vi "_CmdExe._Test run VI with abort and timeout.vi"() -> ()   [LabVIEW 2018]
panel:
  out "Timed Out":bool
  out "Aborted":bool
  out "error out":errorcluster
  in  "Timeout ms":i32=2000
  in  "Test Start":bool
  in  "stop":bool
  out "Running":bool
  in  "Abort":bool
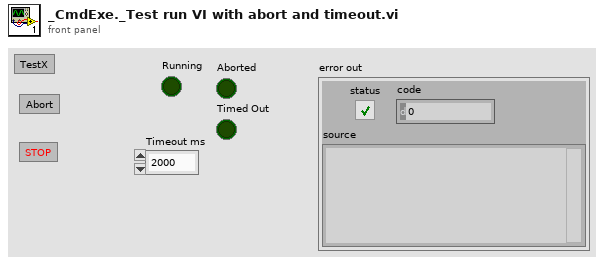
[diagram p1: front panel]
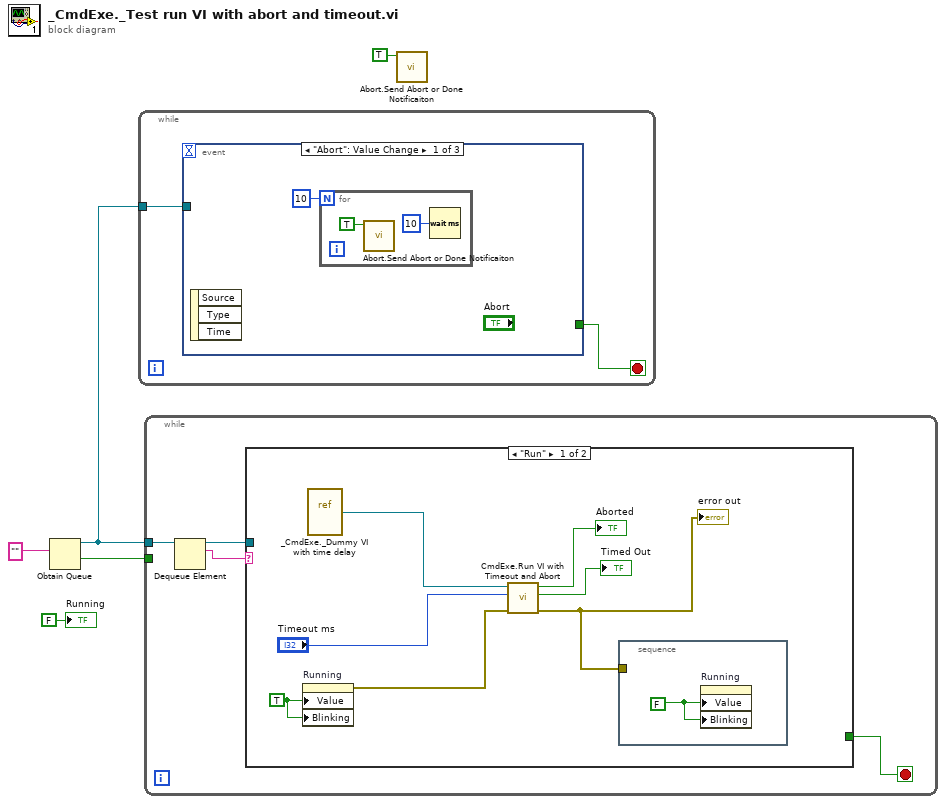
[diagram p0: block diagram]
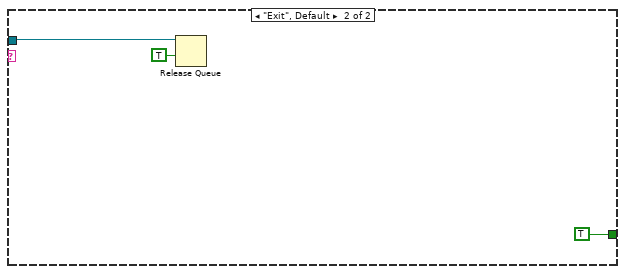
[diagram p2: hidden frame]
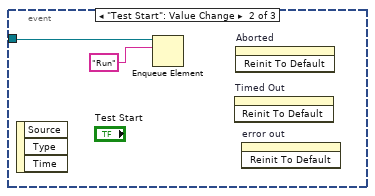
[diagram p3: hidden frame]
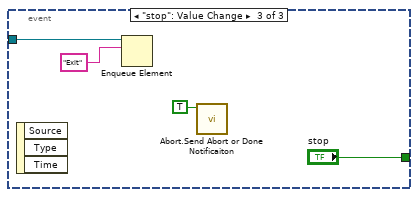
[diagram p4: hidden frame]
diagram:
  n1 = Obtain Queue(element data type="") -> (queue out=w4:refnum<queue>, created new?=w2:bool)  [unwired: 4 in, 1 out]
  n2 = while {
    tunnel: w4 -> [w6]
    stop <- w7 stop-if-true
    n3 = event shown="[0] \"Abort\": Value Change" {
      selector: _ -> [_ _ _]
      dyn-events: _ -> [_ _ _]
      timeout: _ -> [_ _ _]
      tunnel: [_ _ "stop"] -> w7
      tunnel: w6 -> [_ w11 w14]
      event "Abort": Value Change {
        n4 = event-data() -> ()  [unwired: 1 in, 3 out]
        n5 = for {
          N: 10 -> [_]
          n6 = call "Abort.Send Abort or Done Notificaiton.vi"("Abort(T)/Done(F)"=TRUE) -> ()  [unwired: 10 in, 1 out]
          n7 = Wait (ms)(milliseconds to wait=u32 10) -> ()  [unwired: 1 out]
        }
      }
      event "Test Start": Value Change {
        n8 = event-data() -> ()  [unwired: 1 in, 3 out]
        n9 = Enqueue Element(queue=w11, element="Run") -> ()  [unwired: 2 in, 3 out]
        n10 = invoke on="Timed Out" class="Bool (strict)" method="Reinit To Default"() -> ()  [unwired: 3 in, 3 out]
        n11 = invoke on="Aborted" class="Bool (strict)" method="Reinit To Default"() -> ()  [unwired: 3 in, 3 out]
        n12 = invoke on="error out" class="Clust (strict)" method="Reinit To Default"() -> ()  [unwired: 3 in, 3 out]
      }
      event "stop": Value Change {
        n13 = event-data() -> ()  [unwired: 1 in, 3 out]
        n14 = Enqueue Element(queue=w14, element="Exit") -> ()  [unwired: 2 in, 3 out]
        n15 = call "Abort.Send Abort or Done Notificaiton.vi"("Abort(T)/Done(F)"=TRUE) -> ()  [unwired: 10 in, 1 out]
      }
    }
  }
  n16 = while {
    tunnel: w4 -> [w20]
    tunnel: w2 -> [_]
    stop <- w17 stop-if-true
    n17 = Dequeue Element(queue=w20) -> (queue out=w18:refnum<queue>, element=w19:string)  [unwired: 2 in, 2 out]
    n18 = case shown="\"Run\"" w19 {
      tunnel: w18 -> [_ w30]
      tunnel: [_ TRUE] -> w17
      frame "Run" {
        w27 = TRUE
        n19 = property on="Running" class="Bool (strict)"("Value"=w27, "Blinking"=w27) -> (error out=w24:errorcluster)  [unwired: 2 in, 1 out]
        n20 = vi-ref "_CmdExe._Dummy VI with time delay.vi"() -> (w26:refnum<vi>)
        n21 = call "CmdExe.Run VI with Timeout and Abort.vi"("error in (no error)"=w24, "Timeout ms(-1)"="Timeout ms", "VI Refnum"=w26) -> ("error out"=w21:errorcluster, "Timeout"=→"Timed Out":bool, "Abort"=→"Aborted":bool)  [unwired: 6 in]
        "error out" <- w21
        n22 = stacked-sequence {
          tunnel: w21 -> [_]
          frame #0 {
            w28 = FALSE
            n23 = property on="Running" class="Bool (strict)"("Value"=w28, "Blinking"=w28) -> ()  [unwired: 2 in, 2 out]
          }
        }
      }
      frame "Exit", Default {
        n24 = Release Queue(queue=w30, force destroy? (F)=TRUE) -> ()  [unwired: 1 in, 3 out]
      }
    }
  }
  n25 = call "Abort.Send Abort or Done Notificaiton.vi"("Abort(T)/Done(F)"=TRUE) -> ()  [unwired: 10 in, 1 out]
  "Running" <- FALSE ("Running")
